vi "DataTypes.vi"() -> ()   [LabVIEW 2018]
panel:
  out "Error Out":errorcluster
  in  "Error In":errorcluster
  in  "Waveform":waveform(dbl)
  out "Waveform Graph":waveform(dbl)(graph)
  out "Array 2":dbl[](array[numeric])
  in  "Array":dbl[](array[numeric])
  out "String 2":string
  in  "String":string
  out "Boolean 2":bool
  in  "Boolean":bool
  out "Numeric 4":i32
  in  "Numeric 3":i32
  out "Numeric 2":dbl
  in  "Numeric":dbl
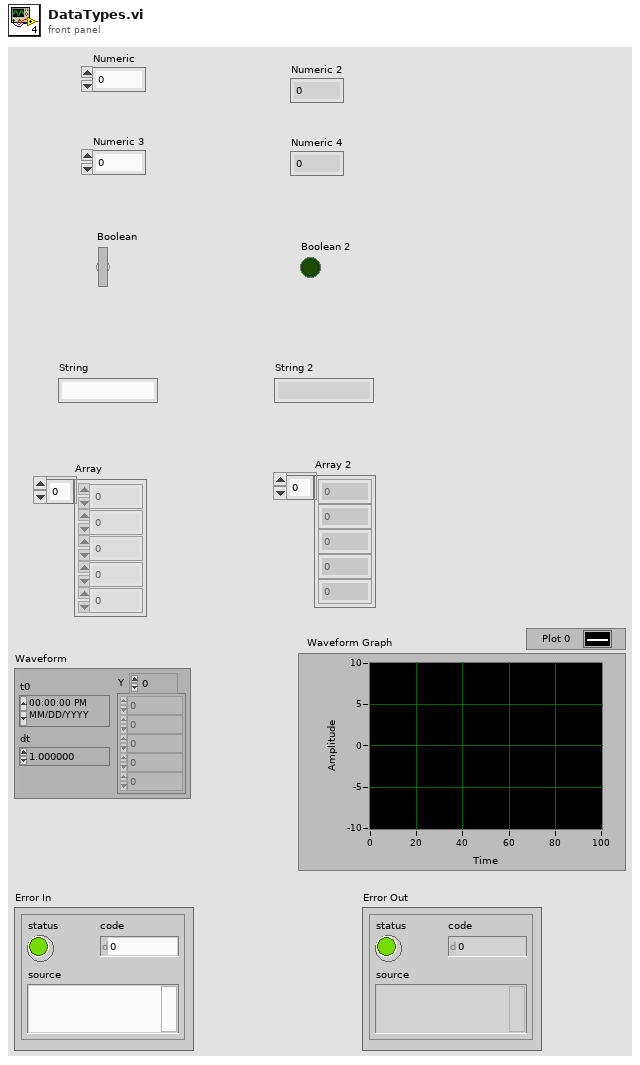
[diagram p1: front panel]
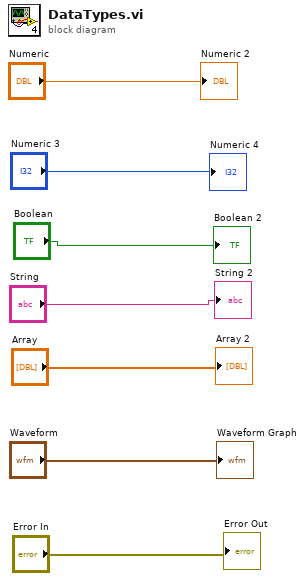
[diagram p0: block diagram]
diagram:
  "Numeric 2" <- "Numeric"
  "Numeric 4" <- "Numeric 3"
  "Boolean 2" <- "Boolean"
  "String 2" <- "String"
  "Array 2" <- "Array"
  "Waveform Graph" <- "Waveform"
  "Error Out" <- "Error In"
